vi "String to Fit Model.vi"(2 "String":string) -> (7 "Fit Model":T1)   [LabVIEW 2021, in "Fits.lvlib"]
uses:
  Fits.lvlib
  Fit Models.ctl
panel:
  in  "Fit Model List":T1=enum."Lorentzian"
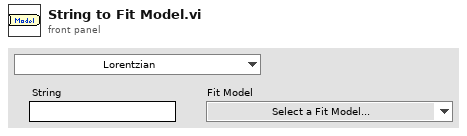
[diagram p1: front panel]
types:
  T1 = typedef "Fits.lvlib/Fit Models.ctl" = enum16{"Select a Fit Model...", "           Single Peak", "Gaussian", "Asymmetric Gaussian", "Lorentzian", "Asymmetric Lorentzian", "Gaussian/Lorentzian", "Lorentzian/Gaussian", "           Double Peak", "Two Gaussians", "Two Asymmetric Gaussians", "Two H-Connected Gaussians", "Two T-Connected Gaussians", "Two H-Connected Asymmetric Gaussians", "Two T-Connected Asymmetric Gaussians", "           Triple Peak", "Three Gaussians", "Three Asymmetric Gaussians", "              Decays", "1-Exponential", "IRF*PSED", "2-Exponentials", "               ACF", "2D Gaussian ACF", "2D Gaussian + Blinking ACF", "2D Gaussian + Flow ACF", "3D Gaussian ACF", "3D Gaussian + Blinking ACF", "             Multiplot", "2D Gaussian ACF & 2D Gaussian + Flow ACF"}
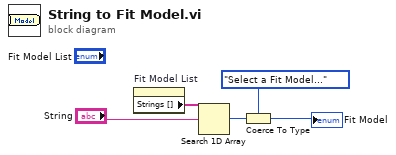
[diagram p0: block diagram]
diagram:
  n1 = property on="Fit Model List" class="Enum (strict)"() -> ("Strings []"=w5:string[])  [unwired: 2 in, 2 out]
  n2 = Search 1D Array(1D array=w5, element="String") -> (index of element=w3:i32)  [unwired: 1 in]
  n3 = Coerce To Type(0:w3, 1:Fit_Models."Select a Fit Model..." ("Fit Model")) -> (2:→"Fit Model":T1)
